vi "Parse TXT Configuration File_Checks.vi"(8 "error in (no error)":errorcluster, 11 "DMAs In":T1[](array[typedef])) -> (0 "error out":errorcluster, 3 "DMAs Out":T1[](array[typedef]))   [LabVIEW 2017, in "GE_RM_System Explorer.lvlib"]
uses:
  GE_RM_System Explorer.lvlib
  Typedef_DMA Instance.ctl
  Typedef_DMA Block Settings.ctl
  Shared/Data Channel Type.ctl
  Typedef_Channel Settings.ctl
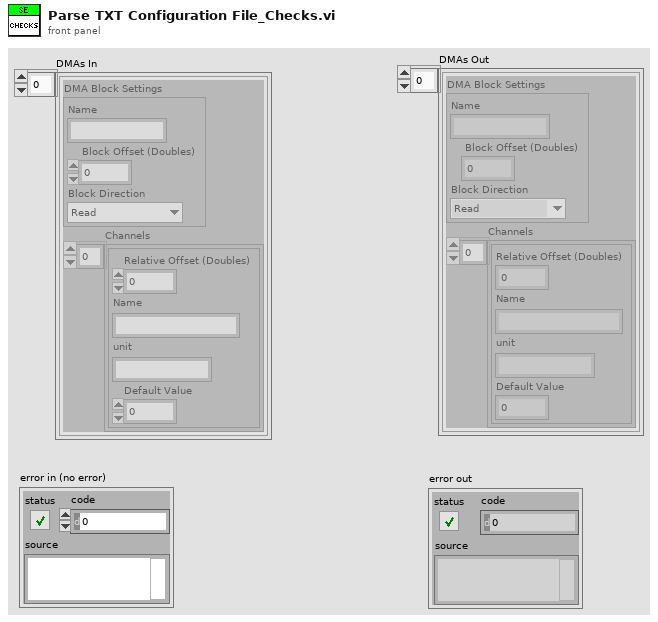
[diagram p1: front panel]
types:
  T1 = typedef "GE_RM_System Explorer.lvlib/Typedef_DMA Instance.ctl" = cluster{"DMA Block Settings":T2, "Channels":T4[]}
  T2 = typedef "GE_RM_System Explorer.lvlib/Typedef_DMA Block Settings.ctl" = cluster{"Name":string, " Block Offset (Doubles)":u32, "Block Direction":T3}
  T3 = typedef "GE_RM_System Explorer.lvlib/Data Channel Type.ctl" = enum16{"Read", "Write"}
  T4 = typedef "GE_RM_System Explorer.lvlib/Typedef_Channel Settings.ctl" = cluster{"Relative Offset (Doubles)":u32, "Name":string, "unit":string, "Default Value":dbl}
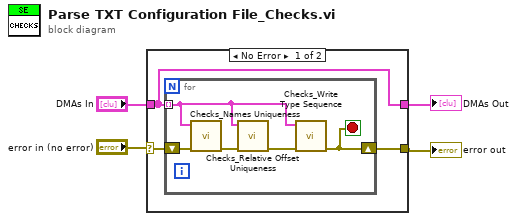
[diagram p0: block diagram]
diagram:
  n1 = case shown="No Error" "error in (no error)" {
    selector: "error in (no error)" -> [w7 w14]
    tunnel: "DMAs In" -> [w5 w13]
    tunnel: [w6 w14] -> w2
    tunnel: [w5 w13] -> w1
    frame No Error {
      n2 = for {
        shift-right: [w8] -> w6
        shift-left: w7 -> [w12]
        tunnel: w5 -> [w9] mode=indexing
        stop <- w8 stop-if-true
        n3 = call "Checks_Names Uniqueness.vi"("error in (no error)"=w12, "DMA"=w9) -> ("error out"=w11:errorcluster)  [unwired: 9 in]
        n4 = call "Checks_Relative Offset Uniqueness.vi"("error in (no error)"=w11, "DMA"=w9) -> ("error out"=w10:errorcluster)  [unwired: 9 in]
        n5 = call "Checks_Write Type Sequence.vi"("error in (no error)"=w10, "DMA"=w9) -> ("error out"=w8:errorcluster)  [unwired: 9 in]
      }
    }
    frame Error {
    }
  }
  "error out" <- w2
  "DMAs Out" <- w1
